vi "Get MSS.vi"(8 "error in (no error)":errorcluster, 11 "Task Base in":refnum<class "Task Base.lvclass">) -> (0 "error out":errorcluster, 2 "MSS":refnum<class "Measure and Stimulus Subsystems.lvclass">, 3 "Task Base out":refnum<class "Task Base.lvclass">)   [LabVIEW 2023, in "Task Base.lvclass"]
uses:
  Task Base.lvclass
  Measure and Stimulus Subsystems/Measure and Stimulus Subsystems.lvclass
  Task Base.lvclass/Task Base.ctl
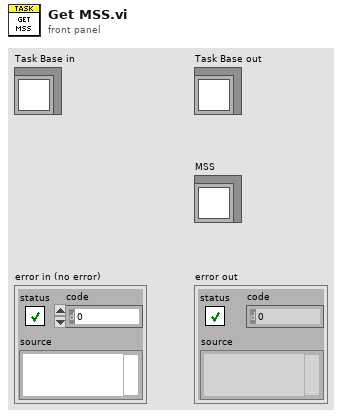
[diagram p1: front panel]
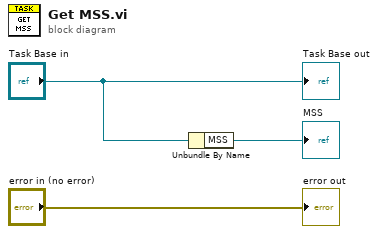
[diagram p0: block diagram]
diagram:
  n1 = Unbundle By Name("Task Base in") -> ("MSS"=→"MSS":refnum<class "Measure and Stimulus Subsystems.lvclass">)
  "error out" <- "error in (no error)"
  "Task Base out" <- "Task Base in"
